vi "sc5511a_soft_front_panel.vi"() -> ()   [LabVIEW 2010]
panel:
  out "message":string="List/Sweep Mode Disabled"
  out "Selected Resource":string
  out "On":bool
  in  "stop":bool
  in  "Tab Control":T1(tab)
  in  "Phase":sgl min=-720 max=720 step=0.1 format="%.1f"
  in  "Spur Suppression":u8(ring) items=["Enabled", "Disabled"]
  in  "AutoLevel":u8(ring) items=["Enable", "Disable"]
  in  "Loop Gain":u8(ring) items=["Normal", "Low"]
  in  "Ref. Out Freq":u8(ring) items=["10 MHz", "100 MHz"]
  in  "Ref. Clock Source":u8(ring) items=["Internal 10 MHz", "Lock to External"]
  in  "RF1 Standby":bool
  in  "Lock Mode":u8(ring) items=["Harmonic Lock", "Frac-N Lock"]
  in  "ALC MODE":u8(ring) items=["Closed", "Opened"]
  in  "Power":sgl=30.0 min=-40 max=30 format="%.2f"
  in  "Interval (s)":u16=5
  in  "GetStatus":bool
  in  "Trigger":bool
  out "Device Status":T2={"Synth Mode"=1, "RF Out"=0, "Auto Level"=0, "ALC Mode"=1, "Standby"=1, "Rf RF Mode"=0, "List Mode State"=0, "RF2 Standby"=0, "Ref Lock Enable"=1, "Ext Ref Detected"=1, "Ref out mode"=1, "Main PLL"=1, "Crs PLL"=1, "Fine PLL"=1, "device accessed"=0, "Over Temp"=0, "MainLED"=FALSE, "CrsLED"=FALSE, "FineLED"=FALSE} {"Over Temp" items=["Normal", "Over Temp"]; "Ref out mode" items=["10 MHz", "100 MHz"]; "device accessed" items=["NO", "YES"]; "RF2 Standby" items=["Disabled", "Enabled"]; "Standby" items=["Disable", "Enabled"]; "Auto Level" items=["Enable", "Disable"]; "Ext Ref Detected" items=["Not Detected", "Detected"]; "Ref Lock Enable" items=["Disabled", "Enabled"]; "RF Out" items=["Disabled", "Enabled"]; "ALC Mode" items=["Closed", "Opened"]; "Rf RF Mode" items=["Single Tone", "List/Sweep"]; "Synth Mode" items=["Harmonic", "FracN"]; "List Mode State" items=["Not Triggered", "Triggered"]; "Main PLL" items=["NOT Locked", "Locked"]; "Crs PLL" items=["NOT Locked", "Locked"]; "Fine PLL" items=["NOT Locked", "Locked"]}
  in  "RF Frequency":dbl=2005000000.0 min=80000000.0 max=21000000000.0 step=1.0 format="%.9p"
  in  "RF Mode":u8(ring) items=["Single Tone", "List/Sweep"]
  in  "RF Enable":bool
  in  "RF2 Freq":sgl=6000.0 min=25 max=6000 step=25
  in  "RF2 Standby":bool
  in  "Set As Default":bool
  in  "Dwell Period (ms)":dbl=10.0 min=0.0 step=0.5 format="%.1f"
  in  "Sweep/List Cycles":u32
  in  "Sweep Freq Parameter":T3={"Start Frequency"=10040000000, "Stop Frequency"=10050000000, "Step Frequency"=100000} {"Step Frequency" max=6500000000 format="%.9p"; "Stop Frequency" max=21000000000 format="%.9p"; "Start Frequency" format="%.9p"}
  in  "List Mode Config":T4={"Sweep / List"=1, "Direction"=0, "Shape"=1, "Trigger Source"=1, "HW Trigger Mode"=0, "Return to Start"=0, "Trigger Out State"=1, "Trigger Out Behavior"=0} {"Trigger Out Behavior" items=["Trigger On Step", "Trigger On Cycle"]; "Trigger Out State" items=["Trigger Out Disable", "Trigger Out Enable"]; "Return to Start" items=["Stop at End", "Return to Start"]; "HW Trigger Mode" items=["Start/Stop", "Step"]; "Trigger Source" items=["Software", "Hardware"]; "Shape" items=["Sawtooth", "Triangle"]; "Direction" items=["Low to High", "High to Low"]; "Sweep / List" items=["List", "Sweep (start/stop/step)"]}
  in  "Load Config":bool
  in  "Save Buffer to EEPROM":bool
  in  "Read EEPROM to Buffer":bool
  in  "Download to Buffer":bool
  in  "Read From File":bool
  in  "Frequency List (2048 max)":u64[](array[numeric]) format="%.9p"
  out "message 2":string
  out "List Points":u32
  in  "SelfCal":bool
  out "Temperature":sgl=40.0 min=-30 max=120 format="%.1f"
  out "Device Info":T5={"Product SN"=268435879, "Hardware Rev"=2.0, "Firmware Rev"=2.0, "Manuf Date"={"Year"=14, "Month"=9, "Day"=10, "Hour"=10}} {"Firmware Rev" format="%.2g"; "Hardware Rev" format="%.2g"; "Product SN" format="%.0x"}
  out "error out":errorcluster
  # "(Deg)"
  # "MHz"
  # "Program will stop and the device will \nreinitialize after self calibration"
  # "DegC"
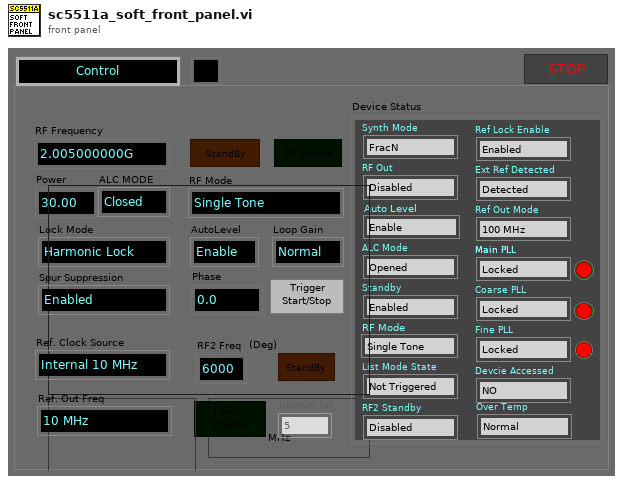
[diagram p1: front panel]
types:
  T1 = enum32{"Control", "Config Sweep/List", "List Entry", "Device Info"}
  T2 = cluster{"Synth Mode":u16, "RF Out":u16, "Auto Level":u16, "ALC Mode":u16, "Standby":u16, "Rf RF Mode":u16, "List Mode State":u16, "RF2 Standby":u16, "Ref Lock Enable":u16, "Ext Ref Detected":u16, "Ref out mode":u16, "Main PLL":u8, "Crs PLL":u8, "Fine PLL":u8, "device accessed":u16, "Over Temp":u16, "MainLED":bool, "CrsLED":bool, "FineLED":bool}
  T3 = cluster{"Start Frequency":u64, "Stop Frequency":u64, "Step Frequency":u64}
  T4 = cluster{"Sweep / List":u8, "Direction":u8, "Shape":u8, "Trigger Source":u8, "HW Trigger Mode":u8, "Return to Start":u8, "Trigger Out State":u8, "Trigger Out Behavior":u8}
  T5 = cluster{"Product SN":u32, "Hardware Rev":sgl, "Firmware Rev":sgl, "Manuf Date":cluster{"Year":u8, "Month":u8, "Day":u8, "Hour":u8}}
  T6 = cluster{"Product SN":u32, "Hardware Rev":sgl, "Firmware Rev":sgl, "Manuf Date":cluster{"Year":u32, "Month":u32, "Day":u32, "hour":u32}}
  T7 = enum32{"Control", "Config Sweep/List", "List Entry"}
  T8 = enum8{"Enabled", "Disabled", "Disabled and Grayed Out"}
  T9 = cluster{"Synth Mode":u16, "RF Out":u16, "Auto Power":u16, "ALC Mode":u16, "Standby":u16, "Rf RF Mode":u16, "List Mode State":u16, "RF2 Standby":u16, "Ref Lock Enable":u16, "Ext Ref Detected":u16, "Ref out mode":u16, "Main PLL":u8, "Crs PLL":u8, "Fine PLL":u8, "device accessed":u16, "Over Temp":u16, "MainLED":bool, "CrsLED":bool, "FineLED":bool}
  T10 = cluster{"Product SN":u32, "Hardware Rev":sgl, "Firmware Rev":sgl, "Manufacture Date":cluster{"Year":u8, "Month":u8, "Day":u8, "hour":u8}}
  T11 = cluster{"List Mode Config":cluster{"List/SSS":u8, "Direction":u8, "Shape":u8, "Trigger Source":u8, "HW Trigger Mode":u8, "Return to Start":u8, "Trigger Out State":u8, "Trigger Out Behavior":u8}, "Operate Status":cluster{"Lock Mode":u8, "Loop Gain":u8, "Device Accessed":u8, "RF2 Standby":u8, "RF1 Standby":u8, "AutoPwrLevel":u8, "AlcMode":u8, "RFOutState":u8, "Ref Lock Enable":u8, "ExtRefDetected":u8, "RefOutSelect":u8, "ListRuning":u8, "RF Mode":u8, "OverTempStatus":u8, "Harmonic_SS":u8}, "PLL Status":cluster{"Sum PLL":u8, "Crs PLL":u8, "Fine PLL":u8, "Crs Ref PLL":u8, "Crs assist PLL":u8, "Ref Clk PLL":u8, "Clk 10 PLL":u8, "Lo2 PLL":u8}}
  T12 = cluster{"RF1 Freq":u64, "Sweep Start Freq":u64, "Sweep Stop Freq":u64, "Sweep Step Freq":u64, "Sweep dwell time (.5ms)":u32, "Sweep Cycles":u32, "List Buffer Points":u32, "RF1 Level (dBm)":sgl, "RF2 freq":u16}
  T13 = cluster{"List/SSS":u8, "Direction":u8, "Shape":u8, "Trigger Source":u8, "HW Trigger Mode":u8, "Return to Start":u8, "Trigger Out State":u8, "Trigger Out Behavior":u8}
  T14 = cluster{"Sweep Start Freq":u64, "Sweep Stop Freq":u64, "Sweep Step Freq":u64}
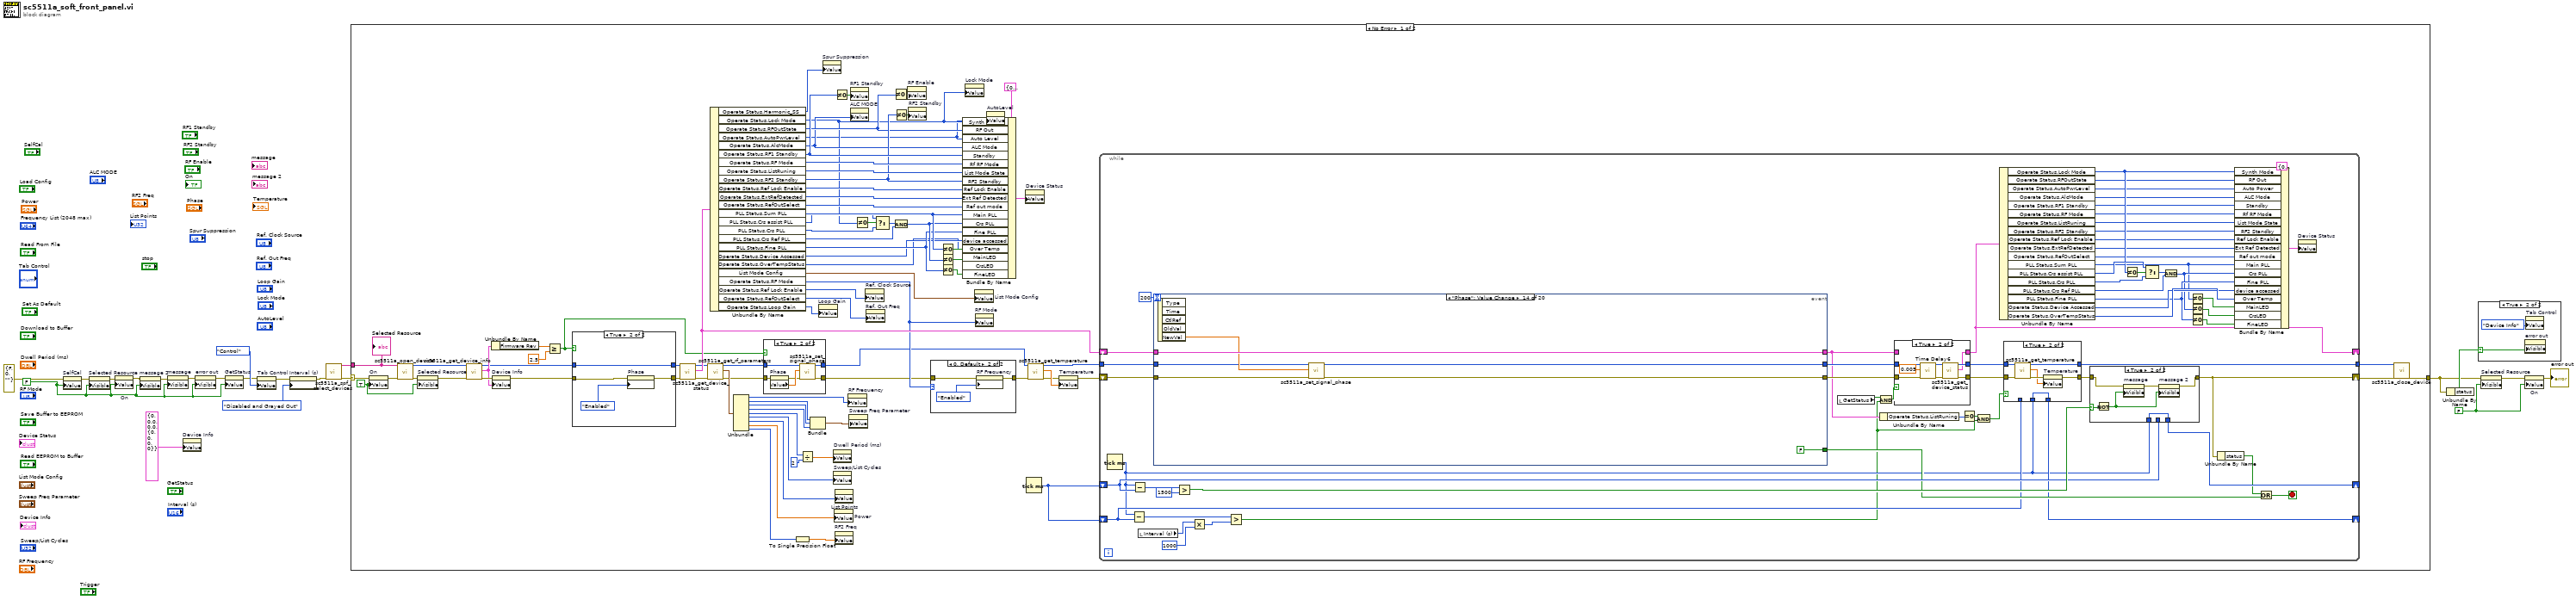
[diagram p0: block diagram]
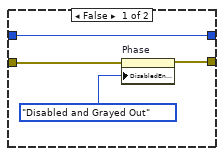
[diagram p3: hidden frame]
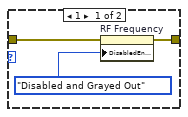
[diagram p5: hidden frame]
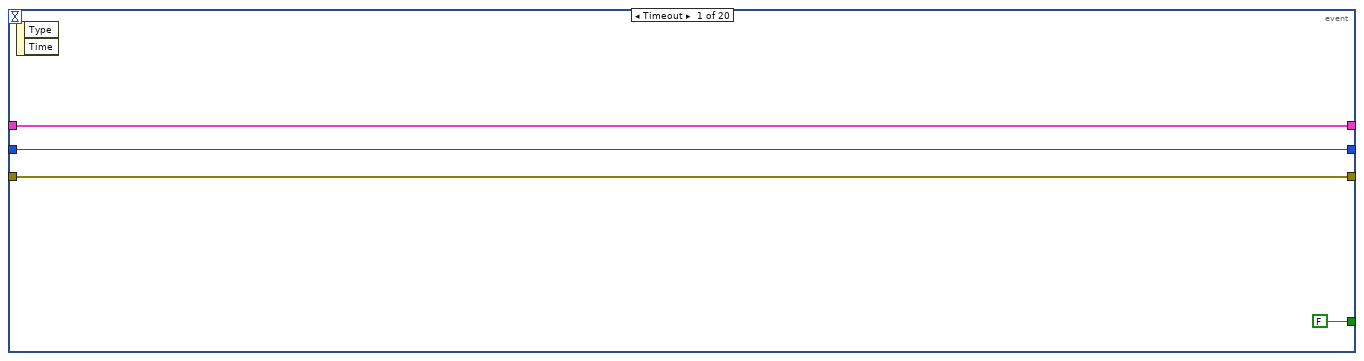
[diagram p9: hidden frame]
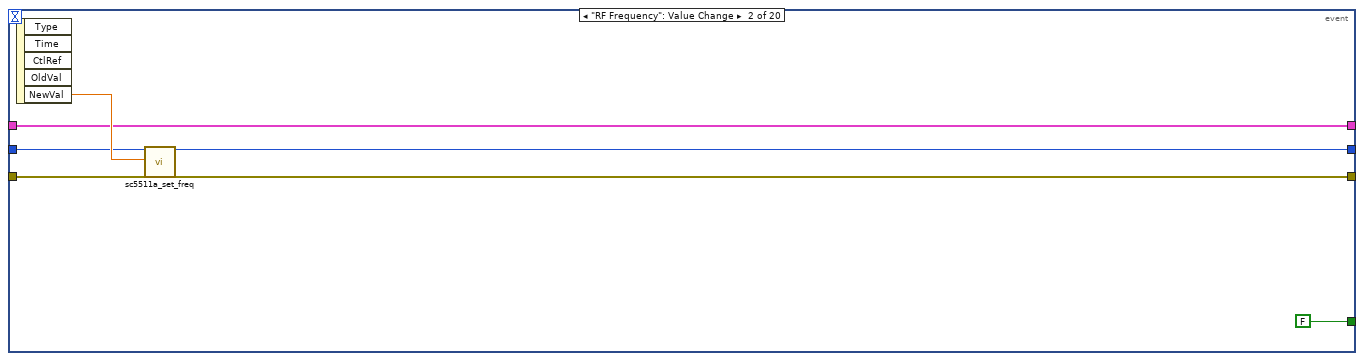
[diagram p10: hidden frame]
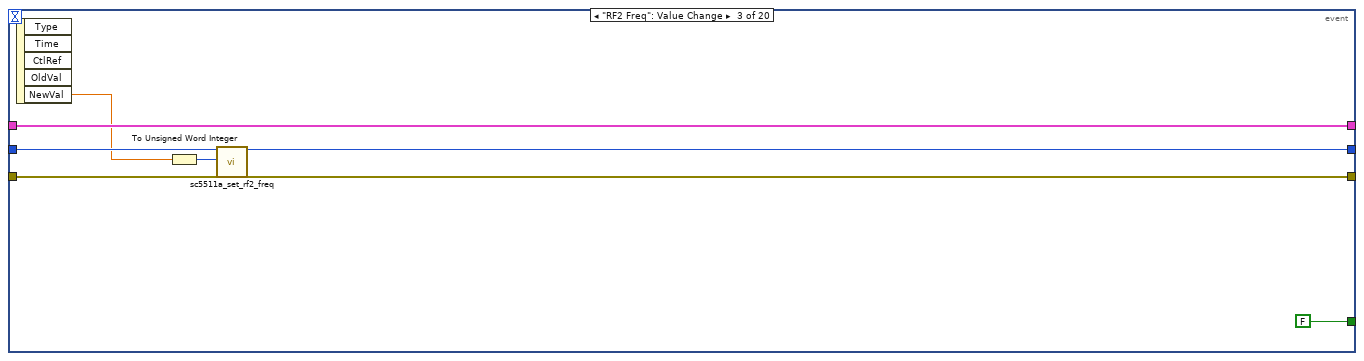
[diagram p11: hidden frame]
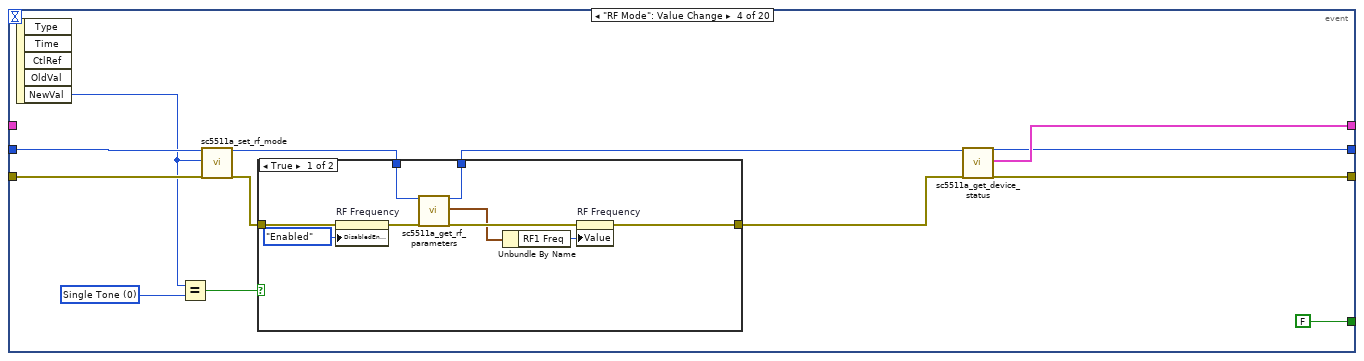
[diagram p12: hidden frame]
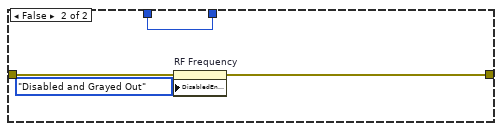
[diagram p13: hidden frame]
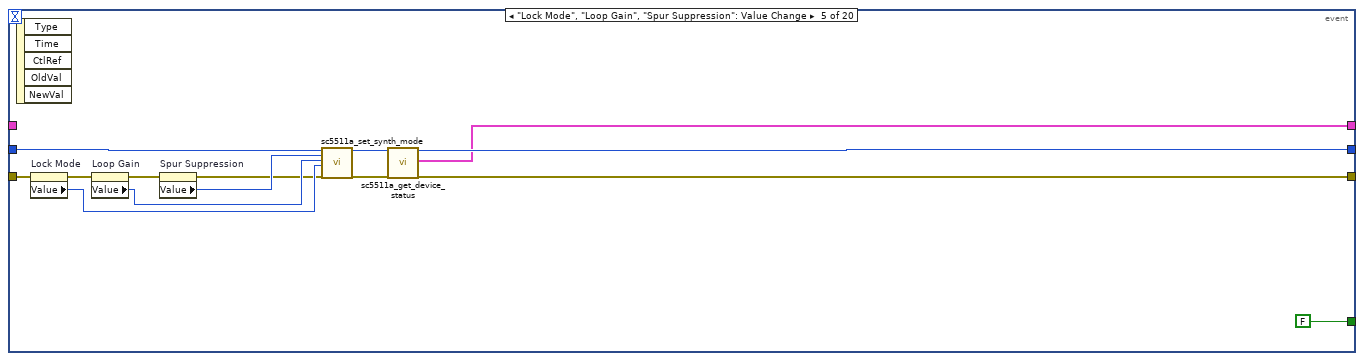
[diagram p14: hidden frame]
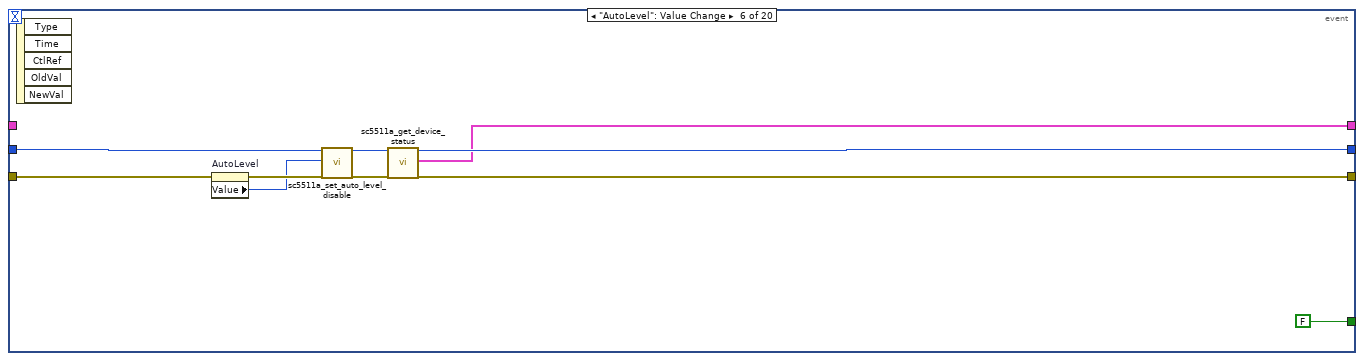
[diagram p15: hidden frame]
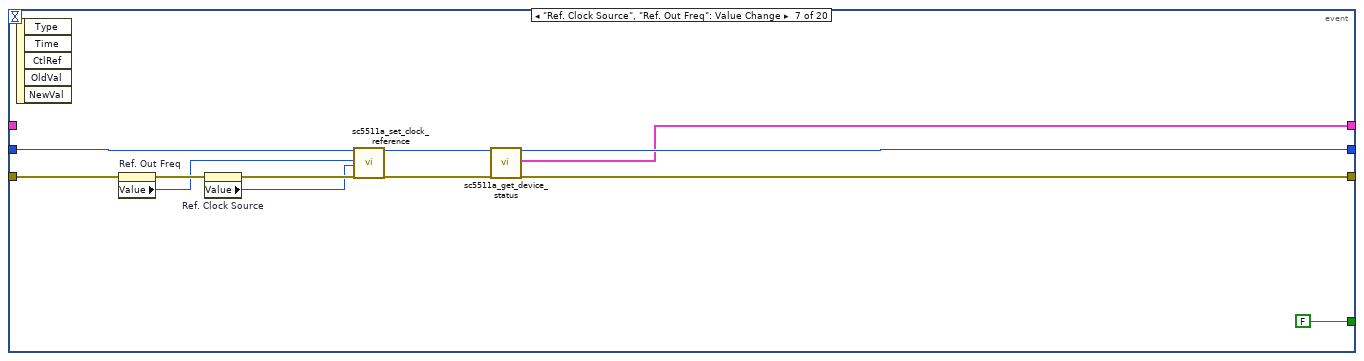
[diagram p16: hidden frame]
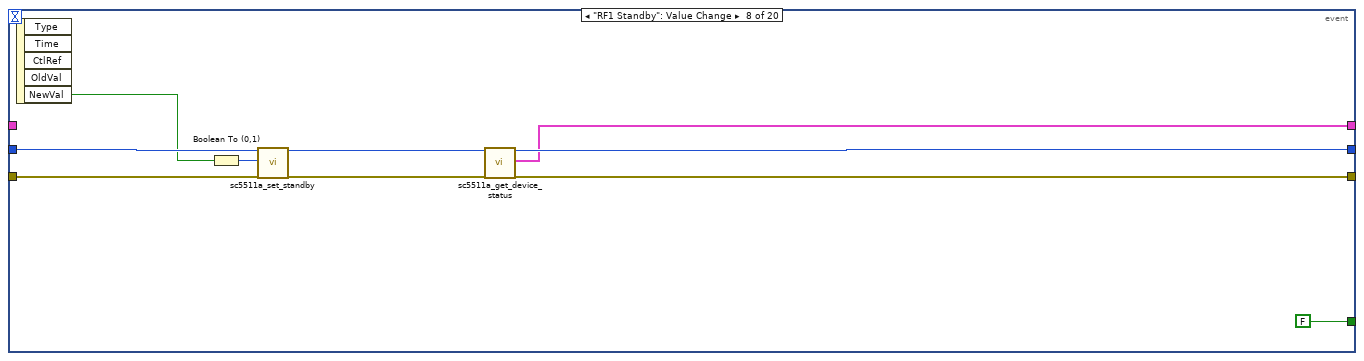
[diagram p17: hidden frame]
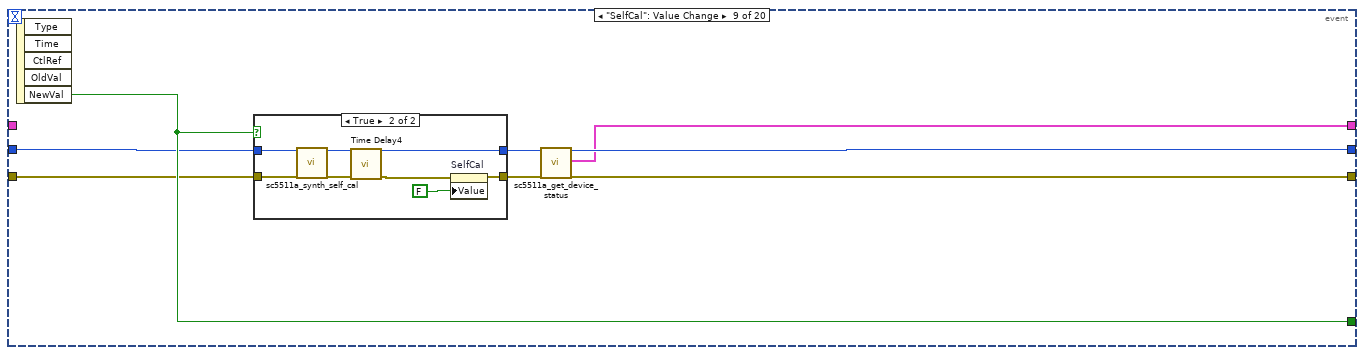
[diagram p18: hidden frame]
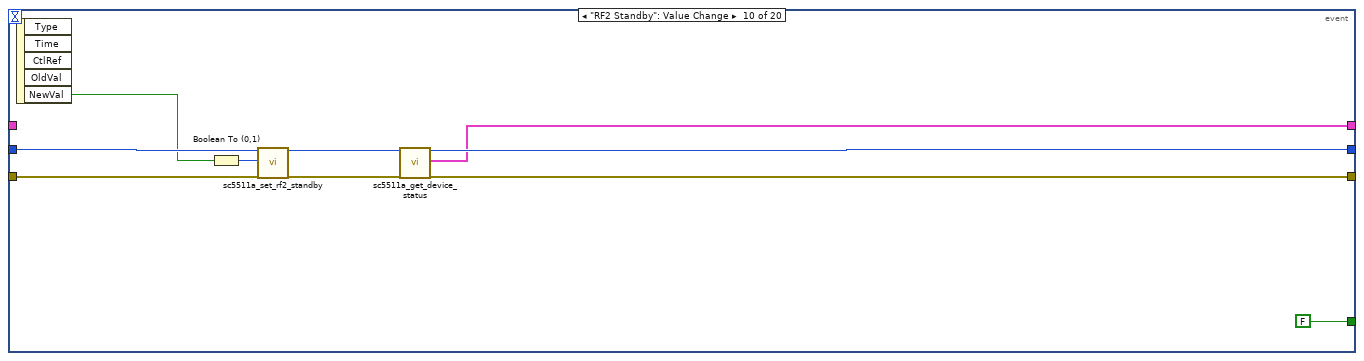
[diagram p20: hidden frame]
diagram:
  w4 = FALSE ("Visible")
  w2 = FALSE ("Visible")
  n1 = property on="SelfCal" class="Bool (strict)"(error in=errorcluster {"status"=FALSE, "code"=0, "source"=""} ("error in (no error)"), "Value"=w2) -> (error out=w3:errorcluster)  [unwired: 1 in, 1 out]
  n2 = property on="Selected Resource" class="Str"(error in=w3, "Visible"=w2) -> (error out=w7:errorcluster)  [unwired: 1 in, 1 out]
  n3 = property on="On" class="Bool (strict)"(error in=w7, "Value"=w2) -> (error out=w12:errorcluster)  [unwired: 1 in, 1 out]
  n4 = property on="message 2" class="Str"(error in=w12, "Visible"=w2) -> (error out=w21:errorcluster)  [unwired: 1 in, 1 out]
  n5 = property on="message" class="Str"(error in=w21, "Visible"=w2) -> (error out=w20:errorcluster)  [unwired: 1 in, 1 out]
  n6 = property on="Device Info" class="Clust (strict)"("Value"=T6 {"Product SN"=0, "Hardware Rev"=0.0, "Firmware Rev"=0.0, "Manuf Date"={"Year"=0, "Month"=0, "Day"=0, "hour"=0}} ("Device Info")) -> ()  [unwired: 2 in, 2 out]
  n7 = property on="error out" class="Clust (strict)"(error in=w20, "Visible"=w2) -> (error out=w19:errorcluster)  [unwired: 1 in, 1 out]
  n8 = property on="GetStatus" class="Bool (strict)"(error in=w19, "Value"=w2) -> (error out=w15:errorcluster)  [unwired: 1 in, 1 out]
  n9 = property on="Tab Control" class="TabCtl (strict)"(error in=w15, "Value"=T7."Control" ("Tab Control")) -> (error out=w16:errorcluster)  [unwired: 1 in, 1 out]
  n10 = property on="Interval (s)" class="DigNum (strict)"(error in=w16, "DisabledEnum"=T8."Disabled and Grayed Out" ("Disabled")) -> (error out=w9:errorcluster)  [unwired: 1 in, 1 out]
  n11 = call "sc5511a_spf_select_devices.vi"("error in (no error)"=w9) -> ("Selected Resource"=w8:string, "error out"=w10:errorcluster)  [unwired: 17 in]
  n12 = case shown="No Error" w10 {
    selector: w10 -> [w89 w586]
    tunnel: [w100 w586] -> w6
    tunnel: w8 -> [w88 _]
    frame No Error {
      w35 = TRUE ("Visible")
      n13 = property on="On" class="Bool (strict)"(error in=w89, "Value"=w35) -> (error out=w90:errorcluster)  [unwired: 1 in, 1 out]
      n14 = call "sc5511a_open_device.vi"("COM (String) eg COM1"=w88, "error in (no error)"=w90) -> ("deviceHandle"=w92:u32, "error out"=w37:errorcluster)  [unwired: 16 in]
      n15 = property on="Selected Resource" class="Str"(error in=w37, "Visible"=w35) -> (error out=w36:errorcluster)  [unwired: 1 in, 1 out]
      n16 = call "sc5511a_get_device_info.vi"("deviceHandle"=w92, "error in"=w36) -> ("deviceHandle"=w26:u32, "Device Info"=w27:T10, "error out"=w97:errorcluster)  [unwired: 15 in]
      n17 = Unbundle By Name(w27) -> ("Firmware Rev"=w29:sgl)
      n18 = property on="Device Info" class="Clust (strict)"(error in=w97, "Value"=w27) -> (error out=w24:errorcluster)  [unwired: 1 in, 1 out]
      n19 = Greater Or Equal?(x=w29, y=sgl 2.5) -> (x >= y?=w22:bool)
      n20 = case shown="True" w22 {
        tunnel: [w106 w109] -> w23
        tunnel: w24 -> [w103 w108]
        tunnel: w26 -> [w104 w110]
        tunnel: [w104 w110] -> w25
        frame False {
          n21 = property on="Phase" class="DigNum (strict)"(error in=w103, "DisabledEnum"=T8."Disabled and Grayed Out" ("Disabled")) -> (error out=w106:errorcluster)  [unwired: 1 in, 1 out]
        }
        frame True {
          n22 = property on="Phase" class="DigNum (strict)"(error in=w108, "DisabledEnum"=T8."Enabled" ("Disabled")) -> (error out=w109:errorcluster)  [unwired: 1 in, 1 out]
        }
      }
      n23 = call "sc5511a_get_device_status.vi"("deviceHandle"=w25, "error in"=w23) -> ("deviceHandle"=w86:u32, "Device Status"=w98:T11, "error out"=w87:errorcluster)  [unwired: 15 in]
      n24 = call "sc5511a_get_rf_parameters.vi"("deviceHandle"=w86, "error in"=w87) -> ("deviceHandle"=w31:u32, "RF Params"=w85:T12, "error out"=w30:errorcluster)  [unwired: 15 in]
      n25 = Unbundle By Name(w98) -> ("Operate Status.Harmonic_SS"=w34:u8, "Operate Status.Lock Mode"=w41:u8, "Operate Status.RFOutState"=w49:u8, "Operate Status.AutoPwrLevel"=w38:u8, "Operate Status.AlcMode"=w48:u8, "Operate Status.RF1 Standby"=w54:u8, "Operate Status.RF Mode"=w71:u8, "Operate Status.ListRuning"=w70:u8, "Operate Status.RF2 Standby"=w50:u8, "Operate Status.Ref Lock Enable"=w69:u8, "Operate Status.ExtRefDetected"=w68:u8, "Operate Status.RefOutSelect"=w67:u8, "PLL Status.Sum PLL"=w66:u8, "PLL Status.Crs assist PLL"=w62:u8, "PLL Status.Crs PLL"=w61:u8, "PLL Status.Crs Ref PLL"=w63:u8, "PLL Status.Fine PLL"=w59:u8, "Operate Status.Device Accessed"=w58:u8, "Operate Status.OverTempStatus"=w57:u8, "List Mode Config"=w99:T13, "Operate Status.RF Mode"=w91:u8, "Operate Status.Ref Lock Enable"=w56:u8, "Operate Status.RefOutSelect"=w55:u8, "Operate Status.Loop Gain"=w42:u8)
      n26 = Unbundle(w85) -> ("RF1 Freq"=w84:u64, "Sweep Start Freq"=w82:u64, "Sweep Stop Freq"=w81:u64, "Sweep Step Freq"=w80:u64, "Sweep dwell time (.5ms)"=w77:u32, "Sweep Cycles"=w79:u32, "List Buffer Points"=w75:u32, "RF1 Level (dBm)"=w74:sgl, "RF2 freq"=w72:u16)
      n27 = case shown="True" w22 {
        tunnel: [w111 w118] -> w33
        tunnel: [w112 w117] -> w32
        tunnel: w31 -> [w112 w116]
        tunnel: w30 -> [w111 w113]
        frame False {
        }
        frame True {
          n28 = property on="Phase" class="DigNum (strict)"(error in=w113) -> (error out=w114:errorcluster, "Value"=w115:sgl)  [unwired: 1 in, 1 out]
          n29 = call "sc5511a_set_signal_phase.vi"("deviceHandle"=w116, "phase (deg)"=w115, "error in"=w114) -> ("deviceHandle"=w117:u32, "error out"=w118:errorcluster)  [unwired: 15 in]
        }
      }
      n30 = To Single Precision Float(number=w72) -> (single precision float=w73:sgl)
      n31 = Divide(x=w77, y=u32 2) -> (x/y=w78:dbl)
      n32 = Bundle("Sweep Start Freq"=w82, "Sweep Stop Freq"=w81, "Sweep Step Freq"=w80) -> (w83:T14)  [unwired: 1 in]
      n33 = property on="Loop Gain" class="Ring (strict)"("Value"=w42) -> ()  [unwired: 2 in, 2 out]
      n34 = property on="Spur Suppression" class="Ring (strict)"("Value"=w34) -> ()  [unwired: 2 in, 2 out]
      n35 = property on="Dwell Period (ms)" class="DigNum (strict)"("Value"=w78) -> ()  [unwired: 2 in, 2 out]
      n36 = property on="Sweep/List Cycles" class="DigNum (strict)"("Value"=w79) -> ()  [unwired: 2 in, 2 out]
      n37 = Not Equal To 0?(x=w54) -> (x != 0?=w53:bool)
      n38 = property on="Power" class="DigNum (strict)"("Value"=w74) -> ()  [unwired: 2 in, 2 out]
      n39 = property on="List Points" class="DigNum (strict)"("Value"=w75) -> ()  [unwired: 2 in, 2 out]
      n40 = property on="RF2 Freq" class="DigNum (strict)"("Value"=w73) -> ()  [unwired: 2 in, 2 out]
      n41 = property on="RF Frequency" class="DigNum (strict)"("Value"=w84) -> ()  [unwired: 2 in, 2 out]
      n42 = property on="Sweep Freq Parameter" class="Clust (strict)"("Value"=w83) -> ()  [unwired: 2 in, 2 out]
      n43 = property on="RF1 Standby" class="Bool (strict)"("Value"=w53) -> ()  [unwired: 2 in, 2 out]
      n44 = property on="ALC MODE" class="Ring (strict)"("Value"=w48) -> ()  [unwired: 2 in, 2 out]
      n45 = Not Equal To 0?(x=w41) -> (x != 0?=w65:bool)
      n46 = property on="Ref. Clock Source" class="Ring (strict)"("Value"=w56) -> ()  [unwired: 2 in, 2 out]
      n47 = property on="Ref. Out Freq" class="Ring (strict)"("Value"=w55) -> ()  [unwired: 2 in, 2 out]
      n48 = Select(t=w62, s=w65, f=w61) -> (s? t:f=w64:u8)
      n49 = Not Equal To 0?(x=w49) -> (x != 0?=w52:bool)
      n50 = Not Equal To 0?(x=w50) -> (x != 0?=w51:bool)
      n51 = And(x=w64, y=w63) -> (x .and. y?=w60:u8)
      n52 = property on="RF Enable" class="Bool (strict)"("Value"=w52) -> ()  [unwired: 2 in, 2 out]
      n53 = property on="RF2 Standby" class="Bool (strict)"("Value"=w51) -> ()  [unwired: 2 in, 2 out]
      n54 = case shown="0, Default" w91 {
        tunnel: w33 -> [w120 w123]
        tunnel: [w119 w122] -> w46
        frame 1 {
          n55 = property on="RF Frequency" class="DigNum (strict)"(error in=w120, "DisabledEnum"=T8."Disabled and Grayed Out" ("Disabled")) -> (error out=w119:errorcluster)  [unwired: 1 in, 1 out]
        }
        frame 0, Default {
          n56 = property on="RF Frequency" class="DigNum (strict)"(error in=w123, "DisabledEnum"=T8."Enabled" ("Disabled")) -> (error out=w122:errorcluster)  [unwired: 1 in, 1 out]
        }
      }
      n57 = Not Equal To 0?(x=w66) -> (x != 0?=w95:bool)
      n58 = Not Equal To 0?(x=w60) -> (x != 0?=w94:bool)
      n59 = Not Equal To 0?(x=w59) -> (x != 0?=w93:bool)
      n60 = Bundle By Name(cluster=T2 {"Synth Mode"=0, "RF Out"=1, "Auto Level"=1, "ALC Mode"=0, "Standby"=0, "Rf RF Mode"=0, "List Mode State"=0, "RF2 Standby"=1, "Ref Lock Enable"=0, "Ext Ref Detected"=0, "Ref out mode"=0, "Main PLL"=1, "Crs PLL"=1, "Fine PLL"=1, "device accessed"=1, "Over Temp"=0, "MainLED"=TRUE, "CrsLED"=TRUE, "FineLED"=TRUE} ("Device Status"), "Synth Mode"=w41, "RF Out"=w49, "Auto Level"=w38, "ALC Mode"=w48, "Standby"=w54, "Rf RF Mode"=w71, "List Mode State"=w70, "RF2 Standby"=w50, "Ref Lock Enable"=w69, "Ext Ref Detected"=w68, "Ref out mode"=w67, "Main PLL"=w66, "Crs PLL"=w60, "Fine PLL"=w59, "device accessed"=w58, "Over Temp"=w57, "MainLED"=w95, "CrsLED"=w94, "FineLED"=w93) -> (w40:T2)
      n61 = property on="Lock Mode" class="Ring (strict)"("Value"=w41) -> ()  [unwired: 2 in, 2 out]
      n62 = property on="List Mode Config" class="Clust (strict)"("Value"=w99) -> ()  [unwired: 2 in, 2 out]
      n63 = property on="RF Mode" class="Ring (strict)"("Value"=w91) -> ()  [unwired: 2 in, 2 out]
      n64 = property on="AutoLevel" class="Ring (strict)"("Value"=w38) -> ()  [unwired: 2 in, 2 out]
      n65 = property on="Device Status" class="Clust (strict)"("Value"=w40) -> ()  [unwired: 2 in, 2 out]
      n66 = Tick Count (ms)() -> (millisecond timer value=w96:u32)
      n67 = call "sc5511a_get_temperature.vi"("deviceHandle"=w32, "error in"=w46) -> ("deviceHandle"=w47:u32, "temperature"=w45:sgl, "error out"=w43:errorcluster)  [unwired: 15 in]
      n68 = property on="Temperature" class="DigNum (strict)"(error in=w43, "Value"=w45) -> (error out=w44:errorcluster)  [unwired: 1 in, 1 out]
      n69 = while {
        shift-right: [w166] -> w102
        shift-left: w44 -> [w184]
        tunnel: w47 -> [w183]
        tunnel: [w133] -> w101
        shift-right: [w141] -> _
        shift-left: w98 -> [w180]
        shift-right: [w170] -> _
        shift-left: w96 -> [w169]
        shift-right: [w136] -> _
        shift-left: w96 -> [w137]
        stop <- w165 stop-if-true
        n70 = Tick Count (ms)() -> (millisecond timer value=w135:u32)
        n71 = Subtract(x=w135, y=w137) -> (x-y=w174:u32)
        n72 = Subtract(x=w135, y=w169) -> (x-y=w179:u32)
        n73 = local read "Interval (s)"() -> (w175:u16)
        n74 = event shown="[13] \"Phase\": Value Change" {
          selector: _ -> [_ _ _ _ _ _ _ _ _ _ _ _ _ _ _ _ _ _ _ _]
          dyn-events: _ -> [_ _ _ _ _ _ _ _ _ _ _ _ _ _ _ _ _ _ _ _]
          timeout: 200 -> [_ _ _ _ _ _ _ _ _ _ _ _ _ _ _ _ _ _ _ _]
          tunnel: w183 -> [w215 w222 w231 w242 w270 w280 w292 w301 w307 w328 w337 w347 w353 w360 w365 w386 w397 w469 w484 w531]
          tunnel: w184 -> [w216 w221 w230 w243 w264 w272 w291 w302 w306 w329 w338 w348 w354 w357 w370 w383 w398 w468 w485 w532]
          tunnel: [w215 w219 w228 w234 w267 w277 w283 w296 w310 w324 w333 w342 w352 w359 w366 w386 w390 w445 w483 w526] -> w182
          tunnel: [w216 w220 w229 w235 w269 w279 w286 w297 w311 w325 w335 w344 w351 w358 w367 w384 w392 w443 w482 w527] -> w181
          tunnel: w180 -> [w214 w218 w227 _ _ _ _ _ _ _ _ _ w356 w363 _ w387 w393 w441 w477 w524]
          tunnel: [w214 w218 w227 w237 w265 w275 w282 w294 w309 w321 w331 w340 w356 w363 w364 w387 w388 w441 w477 w524] -> w130
          tunnel: [FALSE ("NewVal") FALSE FALSE FALSE FALSE FALSE FALSE FALSE w308 FALSE FALSE FALSE FALSE FALSE FALSE TRUE ("NewVal") FALSE ("NewVal") FALSE ("NewVal") FALSE ("NewVal") FALSE ("NewVal")] -> w168
          event Timeout {
            n75 = event-data() -> ()  [unwired: 1 in, 2 out]
          }
          event "RF Frequency": Value Change {
            n76 = event-data() -> ("NewVal"=w223:dbl)  [unwired: 1 in, 4 out]
            n77 = call "sc5511a_set_freq.vi"("deviceHandle"=w222, "RF1 frequency"=w223, "error in"=w221) -> ("deviceHandle"=w219:u32, "error out"=w220:errorcluster)  [unwired: 15 in]
          }
          event "RF2 Freq": Value Change {
            n78 = event-data() -> ("NewVal"=w224:sgl)  [unwired: 1 in, 4 out]
            n79 = To Unsigned Word Integer(number=w224) -> (unsigned 16bit integer=w225:u16)
            n80 = call "sc5511a_set_rf2_freq.vi"("deviceHandle"=w231, "RF1 frequency (MHz)"=w225, "error in"=w230) -> ("deviceHandle"=w228:u32, "error out"=w229:errorcluster)  [unwired: 15 in]
          }
          event "RF Mode": Value Change {
            w240 = u8 0 items=["Single Tone", "List/Sweep"] ("RF Mode")
            n81 = event-data() -> ("NewVal"=w239:u8)  [unwired: 1 in, 4 out]
            n82 = Equal?(x=w239, y=w240) -> (x = y?=w238:bool)
            n83 = call "sc5511a_set_rf_mode.vi"("deviceHandle"=w242, "RF Mode"=w239, "error in"=w243) -> ("deviceHandle"=w233:u32, "error out"=w241:errorcluster)  [unwired: 15 in]
            n84 = case shown="True" w238 {
              tunnel: w241 -> [w253 w257]
              tunnel: [w249 w256] -> w236
              tunnel: [w246 w254] -> w232
              tunnel: w233 -> [w245 w254]
              frame True {
                n85 = property on="RF Frequency" class="DigNum (strict)"(error in=w253, "DisabledEnum"=T8."Enabled" ("Disabled")) -> (error out=w251:errorcluster)  [unwired: 1 in, 1 out]
                n86 = call "sc5511a_get_rf_parameters.vi"("deviceHandle"=w245, "error in"=w251) -> ("deviceHandle"=w246:u32, "RF Params"=w248:T12, "error out"=w250:errorcluster)  [unwired: 15 in]
                n87 = Unbundle By Name(w248) -> ("RF1 Freq"=w247:u64)
                n88 = property on="RF Frequency" class="DigNum (strict)"(error in=w250, "Value"=w247) -> (error out=w249:errorcluster)  [unwired: 1 in, 1 out]
              }
              frame False {
                n89 = property on="RF Frequency" class="DigNum (strict)"(error in=w257, "DisabledEnum"=T8."Disabled and Grayed Out" ("Disabled")) -> (error out=w256:errorcluster)  [unwired: 1 in, 1 out]
              }
            }
            n90 = call "sc5511a_get_device_status.vi"("deviceHandle"=w232, "error in"=w236) -> ("deviceHandle"=w234:u32, "Device Status"=w237:T11, "error out"=w235:errorcluster)  [unwired: 15 in]
          }
          event "Lock Mode", "Loop Gain", "Spur Suppression": Value Change {
            n91 = event-data() -> ()  [unwired: 1 in, 5 out]
            n92 = property on="Lock Mode" class="Ring (strict)"(error in=w264) -> (error out=w263:errorcluster, "Value"=w261:u8)  [unwired: 1 in, 1 out]
            n93 = property on="Loop Gain" class="Ring (strict)"(error in=w263) -> (error out=w258:errorcluster, "Value"=w262:u8)  [unwired: 1 in, 1 out]
            n94 = property on="Spur Suppression" class="Ring (strict)"(error in=w258) -> (error out=w259:errorcluster, "Value"=w260:u8)  [unwired: 1 in, 1 out]
            n95 = call "sc5511a_set_synth_mode.vi"("deviceHandle"=w270, "Harmonic Spur Suppression"=w260, "loop gain"=w262, "lock mode"=w261, "error in"=w259) -> ("deviceHandle"=w266:u32, "error out"=w268:errorcluster)  [unwired: 13 in]
            n96 = call "sc5511a_get_device_status.vi"("deviceHandle"=w266, "error in"=w268) -> ("deviceHandle"=w267:u32, "Device Status"=w265:T11, "error out"=w269:errorcluster)  [unwired: 15 in]
          }
          event "AutoLevel": Value Change {
            n97 = event-data() -> ()  [unwired: 1 in, 5 out]
            n98 = property on="AutoLevel" class="Ring (strict)"(error in=w272) -> (error out=w274:errorcluster, "Value"=w273:u8)  [unwired: 1 in, 1 out]
            n99 = call "sc5511a_set_auto_level_disable.vi"("deviceHandle"=w280, "auto leveling"=w273, "error in"=w274) -> ("deviceHandle"=w276:u32, "error out"=w278:errorcluster)  [unwired: 15 in]
            n100 = call "sc5511a_get_device_status.vi"("deviceHandle"=w276, "error in"=w278) -> ("deviceHandle"=w277:u32, "Device Status"=w275:T11, "error out"=w279:errorcluster)  [unwired: 15 in]
          }
          event "Ref. Clock Source", "Ref. Out Freq": Value Change {
            n101 = event-data() -> ()  [unwired: 1 in, 5 out]
            n102 = property on="Ref. Out Freq" class="Ring (strict)"(error in=w291) -> (error out=w290:errorcluster, "Value"=w287:u8)  [unwired: 1 in, 1 out]
            n103 = property on="Ref. Clock Source" class="Ring (strict)"(error in=w290) -> (error out=w289:errorcluster, "Value"=w288:u8)  [unwired: 1 in, 1 out]
            n104 = call "sc5511a_set_clock_reference.vi"("deviceHandle"=w292, "Ref Output"=w287, "Lock external"=w288, "error in"=w289) -> ("deviceHandle"=w284:u32, "error out"=w285:errorcluster)  [unwired: 14 in]
            n105 = call "sc5511a_get_device_status.vi"("deviceHandle"=w284, "error in"=w285) -> ("deviceHandle"=w283:u32, "Device Status"=w282:T11, "error out"=w286:errorcluster)  [unwired: 15 in]
          }
          event "RF1 Standby": Value Change {
            n106 = event-data() -> ("NewVal"=w300:bool)  [unwired: 1 in, 4 out]
            n107 = Boolean To (0,1)(Boolean=w300) -> (0, 1=w299:i16)
            n108 = call "sc5511a_set_standby.vi"("deviceHandle"=w301, "Standby"=w299, "error in"=w302) -> ("deviceHandle"=w295:u32, "error out"=w298:errorcluster)  [unwired: 15 in]
            n109 = call "sc5511a_get_device_status.vi"("deviceHandle"=w295, "error in"=w298) -> ("deviceHandle"=w296:u32, "Device Status"=w294:T11, "error out"=w297:errorcluster)  [unwired: 15 in]
          }
          event "SelfCal": Value Change {
            n110 = event-data() -> ("NewVal"=w308:bool)  [unwired: 1 in, 4 out]
            n111 = case shown="True" w308 {
              tunnel: w307 -> [w313 w319]
              tunnel: w306 -> [w312 w320]
              tunnel: [w313 w317] -> w305
              tunnel: [w312 w316] -> w304
              frame False {
              }
              frame True {
                n112 = call "sc5511a_synth_self_cal.vi"("deviceHandle"=w319, "error in"=w320) -> ("deviceHandle"=w317:u32, "error out"=w318:errorcluster)  [unwired: 16 in]
                n113 = call "Time Delay4"("error in (no error)"=w318) -> ("error out"=w315:errorcluster)  [unwired: 10 in]
                n114 = property on="SelfCal" class="Bool (strict)"(error in=w315, "Value"=FALSE ("SelfCal")) -> (error out=w316:errorcluster)  [unwired: 1 in, 1 out]
              }
            }
            n115 = call "sc5511a_get_device_status.vi"("deviceHandle"=w305, "error in"=w304) -> ("deviceHandle"=w310:u32, "Device Status"=w309:T11, "error out"=w311:errorcluster)  [unwired: 15 in]
          }
          event "RF2 Standby": Value Change {
            n116 = event-data() -> ("NewVal"=w327:bool)  [unwired: 1 in, 4 out]
            n117 = Boolean To (0,1)(Boolean=w327) -> (0, 1=w326:i16)
            n118 = call "sc5511a_set_rf2_standby.vi"("deviceHandle"=w328, "Standby"=w326, "error in"=w329) -> ("deviceHandle"=w323:u32, "error out"=w322:errorcluster)  [unwired: 15 in]
            n119 = call "sc5511a_get_device_status.vi"("deviceHandle"=w323, "error in"=w322) -> ("deviceHandle"=w324:u32, "Device Status"=w321:T11, "error out"=w325:errorcluster)  [unwired: 15 in]
          }
          event "ALC MODE": Value Change {
            n120 = event-data() -> ("NewVal"=w336:u8)  [unwired: 1 in, 4 out]
            n121 = call "sc5511a_set_alc_mode.vi"("deviceHandle"=w337, "alc mode"=w336, "error in"=w338) -> ("deviceHandle"=w332:u32, "error out"=w334:errorcluster)  [unwired: 15 in]
            n122 = call "sc5511a_get_device_status.vi"("deviceHandle"=w332, "error in"=w334) -> ("deviceHandle"=w333:u32, "Device Status"=w331:T11, "error out"=w335:errorcluster)  [unwired: 15 in]
          }
          event "RF Enable": Value Change {
            n123 = event-data() -> ("NewVal"=w345:bool)  [unwired: 1 in, 4 out]
            n124 = Boolean To (0,1)(Boolean=w345) -> (0, 1=w346:i16)
            n125 = call "sc5511a_set_output.vi"("deviceHandle"=w347, "RF Output"=w346, "error in"=w348) -> ("deviceHandle"=w341:u32, "error out"=w343:errorcluster)  [unwired: 15 in]
            n126 = call "sc5511a_get_device_status.vi"("deviceHandle"=w341, "error in"=w343) -> ("deviceHandle"=w342:u32, "Device Status"=w340:T11, "error out"=w344:errorcluster)  [unwired: 15 in]
          }
          event "Power": Value Change {
            n127 = event-data() -> ("NewVal"=w350:sgl)  [unwired: 1 in, 4 out]
            n128 = call "sc5511a_set_level.vi"("deviceHandle"=w353, "level (dBm)"=w350, "error in"=w354) -> ("deviceHandle"=w352:u32, "error out"=w351:errorcluster)  [unwired: 15 in]
          }
          event "Phase": Value Change {
            n129 = event-data() -> ("NewVal"=w361:sgl)  [unwired: 1 in, 4 out]
            n130 = call "sc5511a_set_signal_phase.vi"("deviceHandle"=w360, "phase (deg)"=w361, "error in"=w357) -> ("deviceHandle"=w359:u32, "error out"=w358:errorcluster)  [unwired: 15 in]
          }
          event "GetStatus": Value Change {
            n131 = event-data() -> ("NewVal"=w369:bool)  [unwired: 1 in, 4 out]
            n132 = case shown="True" w369 {
              selector: w369 -> [w375 w378]
              tunnel: w370 -> [w377 w381]
              tunnel: [w372 w380] -> w368
              tunnel: [w375 w378] -> _
              frame True {
                n133 = property on="RF Frequency" class="DigNum (strict)"(error in=w377, "DisabledEnum"=T8."Enabled" ("Disabled")) -> (error out=w373:errorcluster)  [unwired: 1 in, 1 out]
                n134 = property on="Interval (s)" class="DigNum (strict)"(error in=w373, "DisabledEnum"=T8."Enabled" ("Disabled")) -> (error out=w372:errorcluster)  [unwired: 1 in, 1 out]
              }
              frame False {
                n135 = property on="Interval (s)" class="DigNum (strict)"(error in=w381, "DisabledEnum"=T8."Disabled and Grayed Out" ("Disabled")) -> (error out=w380:errorcluster)  [unwired: 1 in, 1 out]
              }
            }
            n136 = call "sc5511a_get_device_status.vi"("deviceHandle"=w365, "error in"=w368) -> ("deviceHandle"=w366:u32, "Device Status"=w364:T11, "error out"=w367:errorcluster)  [unwired: 15 in]
          }
          event "stop": Value Change {
            n137 = event-data() -> ()  [unwired: 1 in, 5 out]
            n138 = property on="stop" class="Bool (strict)"(error in=w383, "Value"=FALSE ("stop")) -> (error out=w384:errorcluster)  [unwired: 1 in, 1 out]
          }
          event "Trigger": Value Change {
            (unwired) u16 0 ("ListMode State")
            n139 = event-data() -> ()  [unwired: 1 in, 5 out]
            n140 = Unbundle By Name(w393) -> ("Operate Status.RF Mode"=w401:u8, "Operate Status.ListRuning"=w400:u8, "List Mode Config.Trigger Source"=w399:u8)
            n141 = case shown="0, Default" w401 {
              tunnel: w400 -> [_ w413]
              tunnel: w399 -> [_ w412]
              tunnel: w398 -> [w404 w411]
              tunnel: [w403 w410] -> w395
              tunnel: w397 -> [w407 w409]
              tunnel: [w407 w408] -> w389
              frame 0, Default {
                n142 = property on="message" class="Str"(error in=w404, "Visible"=TRUE, "Value"="List/Sweep Mode Disabled" ("hwtrigSel'd")) -> (error out=w403:errorcluster)  [unwired: 1 in, 1 out]
              }
              frame 1 {
                n143 = case shown="1" w413 {
                  tunnel: w412 -> [w418 _]
                  tunnel: w411 -> [w417 w430]
                  tunnel: [w416 w429] -> w410
                  tunnel: w409 -> [w415 w431]
                  tunnel: [w414 w428] -> w408
                  frame 0, Default {
                    n144 = case shown="0, Default" w418 {
                      tunnel: [w421 w426] -> w416
                      tunnel: w417 -> [w422 w427]
                      tunnel: w415 -> [w420 w423]
                      tunnel: [w419 w423] -> w414
                      frame 0, Default {
                        n145 = call "sc5511a_list_soft_trigger.vi"("deviceHandle"=w420, "error in"=w422) -> ("deviceHandle"=w419:u32, "error out"=w421:errorcluster)  [unwired: 16 in]
                      }
                      frame 1 {
                        n146 = property on="message" class="Str"(error in=w427, "Visible"=TRUE, "Value"="Requires Hardware Tigger " ("hwtrigSel'd")) -> (error out=w426:errorcluster)  [unwired: 1 in, 1 out]
                      }
                    }
                  }
                  frame 1 {
                    n147 = call "sc5511a_list_soft_trigger.vi"("deviceHandle"=w431, "error in"=w430) -> ("deviceHandle"=w428:u32, "error out"=w429:errorcluster)  [unwired: 16 in]
                  }
                }
              }
            }
            n148 = call "Time Delay"("error in (no error)"=w395) -> ("error out"=w394:errorcluster)  [unwired: 10 in]
            n149 = property on="Trigger" class="Bool (strict)"(error in=w394, "Value"=FALSE ("Soft Tigger")) -> (error out=w391:errorcluster)  [unwired: 1 in, 1 out]
            n150 = call "sc5511a_get_device_status.vi"("deviceHandle"=w389, "error in"=w391) -> ("deviceHandle"=w390:u32, "Device Status"=w388:T11, "error out"=w392:errorcluster)  [unwired: 15 in]
          }
          event "Load Config", "Set As Default": Value Change {
            (unwired) u16 0 ("Direction")
            w442 = FALSE ("Soft Tigger")
            n151 = event-data() -> ()  [unwired: 1 in, 5 out]
            n152 = property on="List Mode Config" class="Clust (strict)"(error in=w468) -> (error out=w467:errorcluster, "Value"=w466:T4)  [unwired: 1 in, 1 out]
            n153 = call "sc5511a_list_mode_config.vi"("deviceHandle"=w469, "List Mode Config"=w466, "error in"=w467) -> ("deviceHandle"=w462:u32, "error out"=w465:errorcluster)  [unwired: 15 in]
            n154 = property on="Sweep Freq Parameter" class="Clust (strict)"(error in=w465) -> (error out=w459:errorcluster, "Value"=w464:T3)  [unwired: 1 in, 1 out]
            n155 = Unbundle(w464) -> ("Start Frequency"=w463:u64, "Stop Frequency"=w456:u64, "Step Frequency"=w455:u64)
            n156 = call "sc5511a_list_start_freq.vi"("deviceHandle"=w462, "List Start frequency"=w463, "error in"=w459) -> ("deviceHandle"=w461:u32, "error out"=w458:errorcluster)  [unwired: 15 in]
            n157 = call "sc5511a_list_stop_freq.vi"("deviceHandle"=w461, "RF frequency"=w456, "error in"=w458) -> ("deviceHandle"=w460:u32, "error out"=w457:errorcluster)  [unwired: 15 in]
            n158 = call "sc5511a_list_step_freq.vi"("deviceHandle"=w460, "List Step Frequency"=w455, "error in"=w457) -> ("deviceHandle"=w449:u32, "error out"=w454:errorcluster)  [unwired: 15 in]
            n159 = property on="Sweep/List Cycles" class="DigNum (strict)"(error in=w454) -> (error out=w452:errorcluster, "Value"=w453:u32)  [unwired: 1 in, 1 out]
            n160 = call "sc5511a_list_cycle_count.vi"("deviceHandle"=w449, "List Cycles"=w453, "error in"=w452) -> ("deviceHandle"=w448:u32, "error out"=w451:errorcluster)  [unwired: 15 in]
            n161 = property on="Dwell Period (ms)" class="DigNum (strict)"(error in=w451) -> (error out=w450:errorcluster, "Value"=w447:dbl)  [unwired: 1 in, 1 out]
            n162 = Multiply(x=w447, y=2.0) -> (x*y=w436:dbl)
            n163 = To Unsigned Long Integer(number=w436) -> (unsigned 32bit integer=w435:u32)
            n164 = call "sc5511a_list_dwell_time.vi"("deviceHandle"=w448, "List Dwell Time"=w435, "error in"=w450) -> ("deviceHandle"=w432:u32, "error out"=w433:errorcluster)  [unwired: 15 in]
            n165 = property on="Set As Default" class="Bool (strict)"(error in=w433) -> (error out=w446:errorcluster, "Value"=w444:bool)  [unwired: 1 in, 1 out]
            n166 = case shown="True" w444 {
              tunnel: w446 -> [w471 w475]
              tunnel: [w471 w474] -> w438
              tunnel: w432 -> [w470 w473]
              tunnel: [w470 w472] -> w445
              frame False {
              }
              frame True {
                n167 = call "sc5511a_store_default_state.vi"("deviceHandle"=w473, "error in"=w475) -> ("deviceHandle"=w472:u32, "error out"=w474:errorcluster)  [unwired: 16 in]
              }
            }
            n168 = call "Time Delay3"("error in (no error)"=w438) -> ("error out"=w437:errorcluster)  [unwired: 10 in]
            n169 = property on="Load Config" class="Bool (strict)"(error in=w437, "Value"=w442) -> (error out=w439:errorcluster)  [unwired: 1 in, 1 out]
            n170 = property on="Set As Default" class="Bool (strict)"(error in=w439, "Value"=w442) -> (error out=w443:errorcluster)  [unwired: 1 in, 1 out]
          }
          event "Download to Buffer": Value Change {
            n171 = event-data() -> ()  [unwired: 1 in, 5 out]
            n172 = Unbundle By Name(w477) -> ("Operate Status.RF Mode"=w476:u8)
            n173 = case shown="0, Default" w476 {
              selector: w476 -> [w486 w522]
              tunnel: w485 -> [w497 w520]
              tunnel: w484 -> [w496 w521]
              tunnel: [w494 w521] -> w483
              tunnel: [w493 w519] -> w479
              tunnel: [w486 w522] -> _
              frame 0, Default {
                # "0xFFFFFFFFFF to end buffer write"
                # "0 to reset the buffer to starting address\nand enable buffer write"
                n174 = call "sc5511a_list_buffer_write.vi"("deviceHandle"=w496, "List Frequency"=u64 0 ("Frequency"), "error in"=w497) -> ("deviceHandle"=w489:u32, "error out"=w492:errorcluster)  [unwired: 15 in]
                n175 = property on="Frequency List (2048 max)" class="Arr (strict)"(error in=w492) -> (error out=w490:errorcluster, "Value"=w491:u64[])  [unwired: 1 in, 1 out]
                n176 = for {
                  tunnel: w491 -> [w503] mode=indexing
                  tunnel: w490 -> [w505]
                  tunnel: w489 -> [w504]
                  tunnel: [w502] -> w487
                  tunnel: [w501] -> w488
                  i -> [w499]
                  stop <- w500 stop-if-true
                  n177 = Greater?(x=w499, y=2048) -> (0:w500:bool)
                  n178 = case shown="False" w500 {
                    tunnel: w505 -> [w514 w516]
                    tunnel: [w509 w516] -> w501
                    tunnel: w504 -> [w513 w515]
                    tunnel: w503 -> [w512 _]
                    tunnel: [w511 w515] -> w502
                    tunnel: w499 -> [w508 _]
                    frame False {
                      n179 = call "sc5511a_list_buffer_write.vi"("deviceHandle"=w513, "List Frequency"=w512, "error in"=w514) -> ("deviceHandle"=w511:u32, "error out"=w510:errorcluster)  [unwired: 15 in]
                      n180 = Increment(x=w508) -> (x+1=w507:i32)
                      n181 = property on="List Points" class="DigNum (strict)"(error in=w510, "Value"=w507) -> (error out=w509:errorcluster)  [unwired: 1 in, 1 out]
                    }
                    frame True {
                    }
                  }
                }
                n182 = call "sc5511a_list_buffer_write.vi"("deviceHandle"=w487, "List Frequency"=u64 1099511627775 ("Frequency"), "error in"=w488) -> ("deviceHandle"=w494:u32, "error out"=w493:errorcluster)  [unwired: 15 in]
              }
              frame 1 {
                n183 = property on="message 2" class="Str"(error in=w520, "Value"="List/Sweep On" ("message 2"), "Visible"=TRUE) -> (error out=w519:errorcluster)  [unwired: 1 in, 1 out]
              }
            }
            n184 = call "Time Delay2"("error in (no error)"=w479) -> ("error out"=w478:errorcluster)  [unwired: 10 in]
            n185 = property on="Download to Buffer" class="Bool (strict)"(error in=w478, "Value"=FALSE ("Download to Buffer")) -> (error out=w482:errorcluster)  [unwired: 1 in, 1 out]
          }
          event "Save Buffer to EEPROM", "Read EEPROM to Buffer": Value Change {
            w528 = FALSE ("Copy EEPROM to Buffer")
            n186 = event-data() -> ()  [unwired: 1 in, 5 out]
            n187 = Unbundle By Name(w524) -> ("Operate Status.RF Mode"=w523:u8)
            n188 = case shown="0, Default" w523 {
              tunnel: w532 -> [w538 w583]
              tunnel: w531 -> [w537 w585]
              tunnel: [w534 w584] -> w530
              tunnel: [w533 w585] -> w526
              frame 0, Default {
                n189 = property on="Read EEPROM to Buffer" class="Bool (strict)"(error in=w538) -> (error out=w535:errorcluster, "Value"=w536:bool)  [unwired: 1 in, 1 out]
                n190 = case shown="True" w536 {
                  tunnel: w537 -> [w553 w579]
                  tunnel: w535 -> [w547 w578]
                  tunnel: [w549 w577] -> w534
                  tunnel: [w551 w576] -> w533
                  frame True {
                    w554 = u16 1 items=["Buffer to EEPROM", "EEPROM to Buffer"] ("List Eeprom Config")
                    n191 = property on="List Points" class="DigNum (strict)"(error in=w547) -> (error out=w546:errorcluster, "Value"=w545:u32)  [unwired: 1 in, 1 out]
                    n192 = call "sc5511a_list_buffer_transfer.vi"("deviceHandle"=w553, "transfer mode"=w554, "error in"=w546) -> ("deviceHandle"=w550:u32, "error out"=w552:errorcluster)  [unwired: 15 in]
                    n193 = call "Time Delay5"("error in (no error)"=w552) -> ("error out"=w539:errorcluster)  [unwired: 10 in]
                    n194 = Greater Than 0?(x=w545) -> (x > 0?=w544:bool)
                    n195 = case shown="True" w544 {
                      tunnel: w539 -> [w557 w567]
                      tunnel: [w559 w566] -> w551
                      tunnel: w550 -> [w559 w565]
                      tunnel: [w557 w564] -> w548
                      tunnel: [u64[] [] w563] -> w543
                      tunnel: w545 -> [_ w562]
                      tunnel: [0 w561] -> w540
                      tunnel: [0 ("length") 1 ("length")] -> w542
                      frame False {
                      }
                      frame True {
                        n196 = while {
                          tunnel: w567 -> [w575]
                          tunnel: [w574] -> w564
                          tunnel: [w573] -> w566
                          tunnel: w565 -> [w572]
                          tunnel: [w571] -> w563 mode=indexing
                          tunnel: w562 -> [w570]
                          tunnel: [w568] -> w561
                          i -> [w568]
                          stop <- w569 continue-if-true
                          n197 = Less?(x=w568, y=w570) -> (x < y?=w569:bool)
                          n198 = call "sc5511a_list_buffer_read.vi"("deviceHandle"=w572, "address"=w568, "error in"=w575) -> ("deviceHandle"=w573:u32, "frequency"=w571:u64, "error out"=w574:errorcluster)  [unwired: 14 in]
                        }
                      }
                    }
                    n199 = Delete From Array(array=w543, length=w542, index=w540) -> (array with subset deleted=w541:u64[])  [unwired: 1 out]
                    n200 = property on="List Points" class="DigNum (strict)"("Value"=w540) -> ()  [unwired: 2 in, 2 out]
                    n201 = property on="Frequency List (2048 max)" class="Arr (strict)"(error in=w548, "Value"=w541) -> (error out=w549:errorcluster)  [unwired: 1 in, 1 out]
                  }
                  frame False {
                    w580 = u16 0 items=["Buffer to EEPROM", "EEPROM to Buffer"] ("List Eeprom Config")
                    n202 = call "sc5511a_list_buffer_transfer.vi"("deviceHandle"=w579, "transfer mode"=w580, "error in"=w578) -> ("deviceHandle"=w576:u32, "error out"=w577:errorcluster)  [unwired: 15 in]
                  }
                }
              }
              frame 1 {
                n203 = property on="message 2" class="Str"(error in=w583, "Value"="List Mode On" ("message 2"), "Visible"=TRUE) -> (error out=w584:errorcluster)  [unwired: 1 in, 1 out]
              }
            }
            n204 = property on="Read EEPROM to Buffer" class="Bool (strict)"(error in=w530, "Value"=w528) -> (error out=w529:errorcluster)  [unwired: 1 in, 1 out]
            n205 = property on="Save Buffer to EEPROM" class="Bool (strict)"(error in=w529, "Value"=w528) -> (error out=w527:errorcluster)  [unwired: 1 in, 1 out]
          }
        }
        n206 = Greater?(x=w179, y=u32 1500) -> (0:w177:bool)
        n207 = Multiply(x=w175, y=u16 1000) -> (x*y=w173:u16)
        n208 = Greater?(x=w174, y=w173) -> (0:w127:bool)
        n209 = local read "GetStatus"() -> (w171:bool)
        n210 = And(x=w171, y=w127) -> (x .and. y?=w125:bool)
        n211 = Unbundle By Name(w130) -> ("Operate Status.ListRuning"=w129:u8)
        n212 = case shown="True" w125 {
          tunnel: w182 -> [w205 w212]
          tunnel: w181 -> [w204 w211]
          tunnel: [w204 w209] -> w132
          tunnel: [w205 w210] -> w134
          tunnel: [w203 w208] -> w141
          tunnel: w130 -> [w203 _]
          frame False {
          }
          frame True {
            n213 = call "Time Delay6"("error in (no error)"=w211, "Delay Time (s)"=0.005) -> ("error out"=w207:errorcluster)  [unwired: 9 in]
            n214 = call "sc5511a_get_device_status.vi"("deviceHandle"=w212, "error in"=w207) -> ("deviceHandle"=w210:u32, "Device Status"=w208:T11, "error out"=w209:errorcluster)  [unwired: 15 in]
          }
        }
        n215 = Equal To 0?(x=w129) -> (x = 0?=w128:bool)
        n216 = And(x=w128, y=w127) -> (x .and. y?=w126:bool)
        n217 = Unbundle By Name(w141) -> ("Operate Status.Lock Mode"=w155:u8, "Operate Status.RFOutState"=w145:u8, "Operate Status.AutoPwrLevel"=w146:u8, "Operate Status.AlcMode"=w147:u8, "Operate Status.RF1 Standby"=w148:u8, "Operate Status.RF Mode"=w149:u8, "Operate Status.ListRuning"=w138:u8, "Operate Status.RF2 Standby"=w150:u8, "Operate Status.Ref Lock Enable"=w151:u8, "Operate Status.ExtRefDetected"=w152:u8, "Operate Status.RefOutSelect"=w153:u8, "PLL Status.Sum PLL"=w154:u8, "PLL Status.Crs assist PLL"=w159:u8, "PLL Status.Crs PLL"=w160:u8, "PLL Status.Crs Ref PLL"=w158:u8, "PLL Status.Fine PLL"=w162:u8, "Operate Status.Device Accessed"=w163:u8, "Operate Status.OverTempStatus"=w164:u8)
        n218 = case shown="True" w126 {
          tunnel: [w187 w194] -> w136
          tunnel: w137 -> [w187 _]
          tunnel: w135 -> [_ w194]
          tunnel: w134 -> [w186 w193]
          tunnel: [w186 w192] -> w133
          tunnel: w132 -> [w185 w191]
          tunnel: [w185 w189] -> w131
          frame False {
          }
          frame True {
            n219 = call "sc5511a_get_temperature.vi"("deviceHandle"=w193, "error in"=w191) -> ("deviceHandle"=w192:u32, "temperature"=w188:sgl, "error out"=w190:errorcluster)  [unwired: 15 in]
            n220 = property on="Temperature" class="DigNum (strict)"(error in=w190, "Value"=w188) -> (error out=w189:errorcluster)  [unwired: 1 in, 1 out]
          }
        }
        n221 = case shown="True" w177 {
          selector: w177 -> [_ w199]
          tunnel: w131 -> [w196 w202]
          tunnel: [w196 w201] -> w166
          tunnel: w169 -> [w195 _]
          tunnel: [w195 w197] -> w170
          tunnel: w135 -> [_ w197]
          frame False {
          }
          frame True {
            n222 = Not(x=w199) -> (.not. x?=w198:bool)
            n223 = property on="message" class="Str"(error in=w202, "Visible"=w198) -> (error out=w200:errorcluster)  [unwired: 1 in, 1 out]
            n224 = property on="message 2" class="Str"(error in=w200, "Visible"=w198) -> (error out=w201:errorcluster)  [unwired: 1 in, 1 out]
          }
        }
        n225 = Not Equal To 0?(x=w155) -> (x != 0?=w156:bool)
        n226 = Select(t=w159, s=w156, f=w160) -> (s? t:f=w157:u8)
        n227 = And(x=w157, y=w158) -> (x .and. y?=w161:u8)
        n228 = Not Equal To 0?(x=w154) -> (x != 0?=w142:bool)
        n229 = Not Equal To 0?(x=w161) -> (x != 0?=w143:bool)
        n230 = Not Equal To 0?(x=w162) -> (x != 0?=w144:bool)
        n231 = Unbundle By Name(w166) -> ("status"=w167:bool)
        n232 = Bundle By Name(cluster=T9 {"Synth Mode"=0, "RF Out"=0, "Auto Power"=0, "ALC Mode"=0, "Standby"=0, "Rf RF Mode"=0, "List Mode State"=0, "RF2 Standby"=0, "Ref Lock Enable"=0, "Ext Ref Detected"=0, "Ref out mode"=0, "Main PLL"=1, "Crs PLL"=1, "Fine PLL"=1, "device accessed"=0, "Over Temp"=0, "MainLED"=FALSE, "CrsLED"=FALSE, "FineLED"=FALSE} ("Device Status"), "Synth Mode"=w155, "RF Out"=w145, "Auto Power"=w146, "ALC Mode"=w147, "Standby"=w148, "Rf RF Mode"=w149, "List Mode State"=w138, "RF2 Standby"=w150, "Ref Lock Enable"=w151, "Ext Ref Detected"=w152, "Ref out mode"=w153, "Main PLL"=w154, "Crs PLL"=w161, "Fine PLL"=w162, "device accessed"=w163, "Over Temp"=w164, "MainLED"=w142, "CrsLED"=w143, "FineLED"=w144) -> (w140:T9)
        n233 = Or(x=w167, y=w168) -> (x .or. y?=w165:bool)
        n234 = property on="Device Status" class="Clust (strict)"("Value"=w140) -> ()  [unwired: 2 in, 2 out]
      }
      n235 = call "sc5511a_close_device.vi"("deviceHandle"=w101, "error in (no error)"=w102) -> ("error out"=w100:errorcluster)  [unwired: 17 in]
      "Selected Resource" <- w88
    }
    frame Error {
    }
  }
  n236 = Unbundle By Name(w6) -> ("status"=w11:bool)
  n237 = case shown="True" w11 {
    selector: w11 -> [_ w587]
    frame False {
    }
    frame True {
      n238 = property on="error out" class="Clust (strict)"("Visible"=w587) -> ()  [unwired: 2 in, 2 out]
      n239 = property on="Tab Control" class="TabCtl (strict)"("Value"=T1."Device Info" ("Tab Control")) -> ()  [unwired: 2 in, 2 out]
    }
  }
  n240 = property on="Selected Resource" class="Str"(error in=w6, "Visible"=w4) -> (error out=w5:errorcluster)  [unwired: 1 in, 1 out]
  n241 = property on="On" class="Bool (strict)"(error in=w5, "Value"=w4) -> (error out=→"error out":errorcluster)  [unwired: 1 in, 1 out]
